vi "hama_orca_acquire.vi"(5 "Save properties":T2, 7 "Acq properties":T1, 8 "error in (no error)":errorcluster {"code" format="%.0x"}, 10 "Camera ON status":bool, 11 "Camera handle in":u32) -> (0 "error out":errorcluster {"code" format="%.0x"}, 1 "Image out":u16[][](array[numeric]), 2 "Camera ON":bool=TRUE, 3 "Camera handle out":u32)   [LabVIEW 2018]
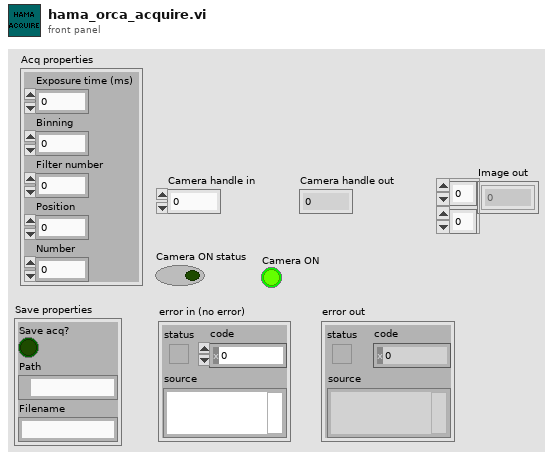
[diagram p1: front panel]
types:
  T1 = cluster{"Exposure time (ms)":dbl, "Binning ":dbl, "Filter number":dbl, "Position":dbl, "Number":i32}
  T2 = cluster{"Save acq?":bool, "Path":path, "Filename":string}
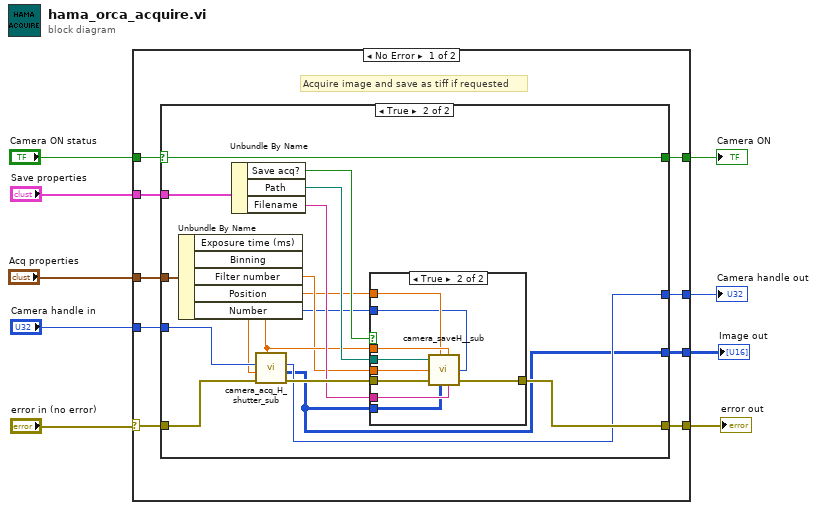
[diagram p0: block diagram]
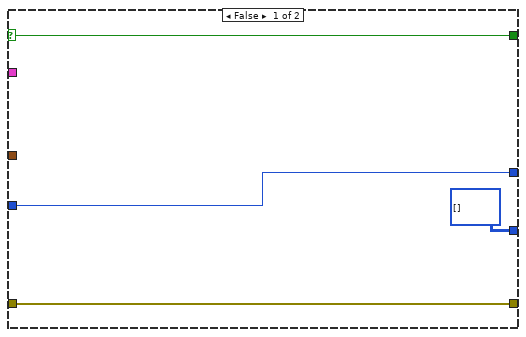
[diagram p2: hidden frame]
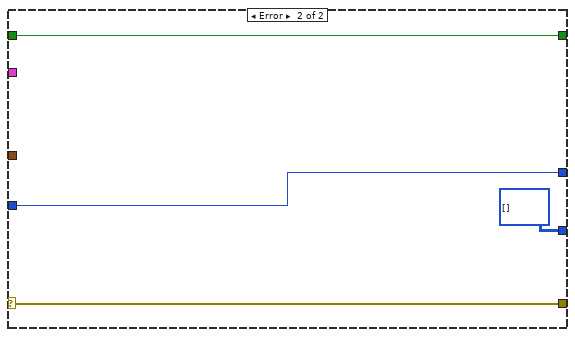
[diagram p4: hidden frame]
diagram:
  n1 = case shown="No Error" "error in (no error)" {
    selector: "error in (no error)" -> [w16 w53]
    tunnel: [w18 w53] -> w9
    tunnel: "Camera ON status" -> [w17 w52]
    tunnel: [w15 w51] -> w6
    tunnel: [w14 w52] -> w5
    tunnel: "Camera handle in" -> [w13 w51]
    tunnel: "Acq properties" -> [w12 _]
    tunnel: "Save properties" -> [w11 _]
    tunnel: [w10 u16[][] [] ("Image")] -> w2
    frame No Error {
      # "Acquire image and save as tiff if requested"
      n2 = case shown="True" w17 {
        selector: w17 -> [w22 w37]
        tunnel: [w20 w28] -> w18
        tunnel: w16 -> [w20 w38]
        tunnel: [w21 w26] -> w15
        tunnel: [w22 w37] -> w14
        tunnel: w13 -> [w21 w39]
        tunnel: w12 -> [_ w36]
        tunnel: w11 -> [_ w34]
        tunnel: [u16[][] [] ("Image") w25] -> w10
        frame False {
        }
        frame True {
          n3 = Unbundle By Name(w36) -> ("Exposure time (ms)"=w29:dbl, "Binning"=w35:dbl, "Filter number"=w27:dbl, "Position"=w24:dbl, "Number"=w23:i32)
          n4 = Unbundle By Name(w34) -> ("Save acq?"=w33:bool, "Path"=w31:path, "Filename"=w30:string)
          n5 = call "camera_acq_H_shutter_sub.vi"("Exposure time (ms)"=w29, "error in (no error)"=w38, "Binning"=w35, "Camera in"=w39) -> ("error out"=w32:errorcluster, "Image"=w25:u16[][], "Camera out"=w26:u32)  [unwired: 5 in]
          n6 = case shown="True" w33 {
            tunnel: w32 -> [w40 w49]
            tunnel: w31 -> [_ w48]
            tunnel: w30 -> [_ w47]
            tunnel: w29 -> [_ w46]
            tunnel: [w40 w45] -> w28
            tunnel: w27 -> [_ w44]
            tunnel: w25 -> [_ w43]
            tunnel: w24 -> [_ w42]
            tunnel: w23 -> [_ w41]
            frame False {
            }
            frame True {
              n7 = call "camera_saveH__sub.vi"("Path"=w48, "Position"=w42, "Filter"=w44, "error in"=w49, "Image"=w43, "Exposure time"=w46, "Number"=w41, "filename"=w47) -> ("error out"=w45:errorcluster)  [unwired: 1 in]
            }
          }
        }
      }
    }
    frame Error {
    }
  }
  "error out" <- w9
  "Camera handle out" <- w6
  "Camera ON" <- w5
  "Image out" <- w2
